vi "Min Dist from Path to Point.vi"(0 "point":cluster{"x":dbl, "y":dbl, "th":dbl}, 1 "Waypoints":cluster{"x":dbl, "y":dbl, "th":dbl}[](array[cluster])) -> (7 "min dist":dbl)   [LabVIEW 2019]
uses:
  <vilib>/Analysis/baseanly.llb/Real Dot Product.vi
  a4369fa1-359a-4df1-a4cd-d76a6dd48147.vi
  <vilib>/Analysis/NI_AALBase.lvlib
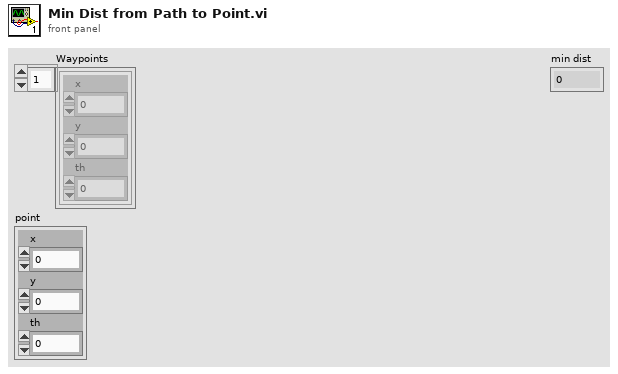
[diagram p1: front panel]
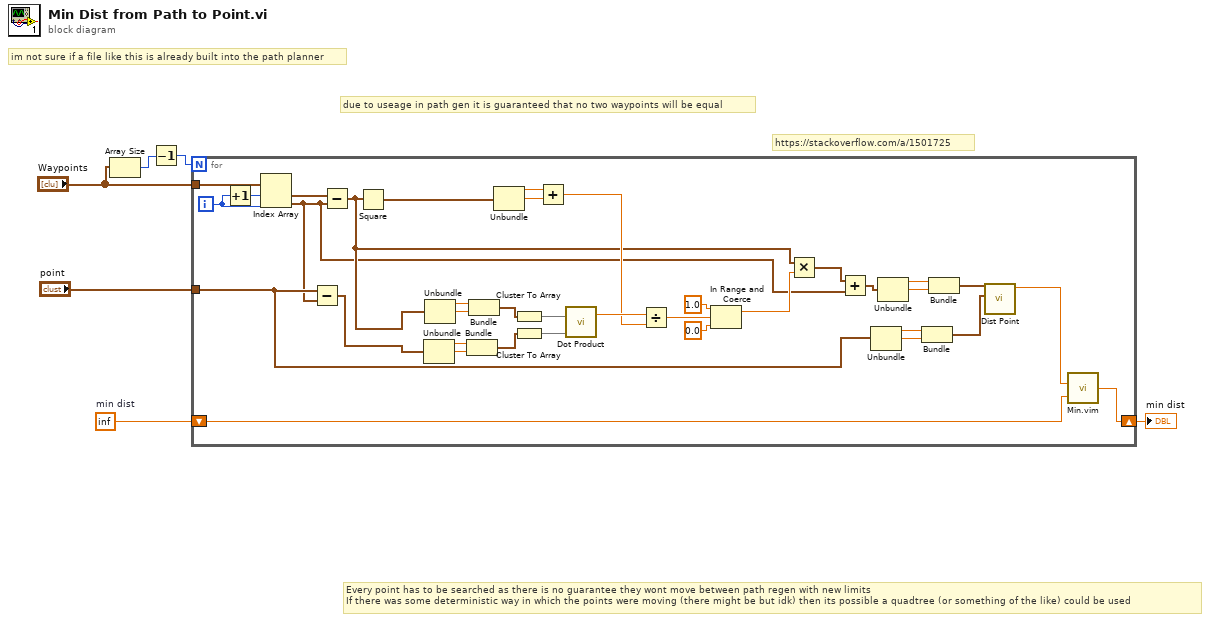
[diagram p0: block diagram]
diagram:
  w5 = inf  # min dist
  # "https://stackoverflow.com/a/1501725"
  # "due to useage in path gen it is guaranteed that no two waypoints will be equal"
  # "Every point has to be searched as there is no guarantee they wont move between path regen with new limits\nIf there was some deterministic way in which the points were moving (there might be but idk) then its possible a quadtree (or something of the like) could be used"
  # "im not sure if a file like this is already built into the path planner"
  n1 = Array Size(array="Waypoints") -> (size(s)=w2:i32)
  n2 = Decrement(x=w2) -> (x-1=w3:i32)
  n3 = for {
    N: w3 -> [_]
    tunnel: "point" -> [w14]
    shift-right: [w9] -> w4
    shift-left: w5 -> [w10]
    tunnel: "Waypoints" -> [w42]
    i -> [w23]
    n4 = Increment(x=w23) -> (x+1=w24:i32)
    n5 = Index Array(array=w42, index #1=w24, index #2=w23) -> (element #1=w21:cluster{"x":dbl, "y":dbl, "th":dbl}, element #2=w7:cluster{"x":dbl, "y":dbl, "th":dbl})
    n6 = Subtract(x=w14, y=w7) -> (x-y=w36:cluster{"x":dbl, "y":dbl, "th":dbl})
    n7 = Subtract(x=w21, y=w7) -> (x-y=w8:cluster{"x":dbl, "y":dbl, "th":dbl})
    n8 = Square(x=w8) -> (x^2=w41:cluster{"x":dbl, "y":dbl, "th":dbl})
    n9 = Unbundle(w36) -> ("x"=w33:dbl, "y"=w32:dbl)  [unwired: 1 out]
    n10 = Unbundle(w8) -> ("x"=w35:dbl, "y"=w34:dbl)  [unwired: 1 out]
    n11 = Bundle("x"=w33, "y"=w32) -> (w30:cluster{"x":dbl, "y":dbl})  [unwired: 1 in]
    n12 = Bundle("x"=w35, "y"=w34) -> (w31:cluster{"x":dbl, "y":dbl})  [unwired: 1 in]
    n13 = Unbundle(w41) -> ("x"=w40:dbl, "y"=w39:dbl)  [unwired: 1 out]
    n14 = Cluster To Array(cluster=w31) -> (array=w38:dbl[])
    n15 = Cluster To Array(cluster=w30) -> (array=w37:dbl[])
    n16 = Add(x=w40, y=w39) -> (x+y=w28:dbl)
    n17 = call-poly <vilib>:"Dot Product.vi"("Y Vector"=w37, "X Vector"=w38) -> ("X * Y"=w29:dbl)  [unwired: 1 out]
    n18 = Divide(x=w29, y=w28) -> (x/y=w27:dbl)
    n19 = In Range and Coerce(upper limit=1.0, x=w27, lower limit=0.0 ("x")) -> (coerced(x)=w22:dbl)  [unwired: 1 out]
    n20 = Multiply(x=w8, y=w22) -> (x*y=w20:cluster{"x":dbl, "y":dbl, "th":dbl})
    n21 = Add(x=w20, y=w7) -> (x+y=w19:cluster{"x":dbl, "y":dbl, "th":dbl})
    n22 = Unbundle(w14) -> ("x"=w12:dbl, "y"=w15:dbl)  [unwired: 1 out]
    n23 = Unbundle(w19) -> ("x"=w18:dbl, "y"=w17:dbl)  [unwired: 1 out]
    n24 = Bundle("x"=w12, "y"=w15) -> (w13:cluster{"x":dbl, "y":dbl})  [unwired: 1 in]
    n25 = Bundle("x"=w18, "y"=w17) -> (w16:cluster{"x":dbl, "y":dbl})  [unwired: 1 in]
    n26 = call "Dist Point.vi"("point b"=w13, "point a"=w16) -> ("dist"=w11:dbl)  [unwired: 9 in]
    n27 = call "Min.vim"("b"=w10, "a"=w11) -> ("min(a, b)"=w9:dbl)
  }
  "min dist" <- w4
